vi "Get SQLite Template Path.vi"(1 "Template Type":T1) -> (0 "Template Path":path)   [LabVIEW 2021]
uses:
  DB Method Enum.ctl
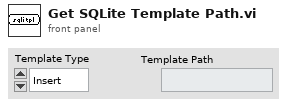
[diagram p1: front panel]
types:
  T1 = typedef "DB Method Enum.ctl" = enum16{"Insert", "Delete", "Select", "Update", "List"}
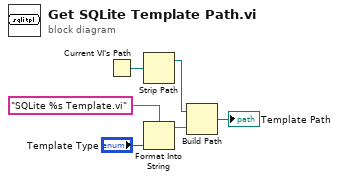
[diagram p0: block diagram]
diagram:
  n1 = Current VI's Path() -> (path=w4:path)
  n2 = Strip Path(path=w4) -> (stripped path=w5:path)  [unwired: 1 out]
  n3 = Format Into String(format string="SQLite %s Template.vi" ("name"), "Template Type") -> (resulting string=w2:string)  [unwired: 2 in, 1 out]
  n4 = Build Path(base path=w5, name or relative path=w2) -> (appended path=→"Template Path":path)
